vi "Configure Bank Definitions.vi"(8 "error in (no error)":errorcluster, 11 "DIG_IO in":refnum<class "DIG_IO.lvclass">) -> (0 "error out":errorcluster, 3 "DIG_IO out":refnum<class "DIG_IO.lvclass">)   [LabVIEW 2019, in "DIG_IO.lvlib" / "DIG_IO.lvclass"]
uses:
  Library/DIG_IO.lvclass
  Library/DIG_IO.lvclass/DIG_IO.ctl
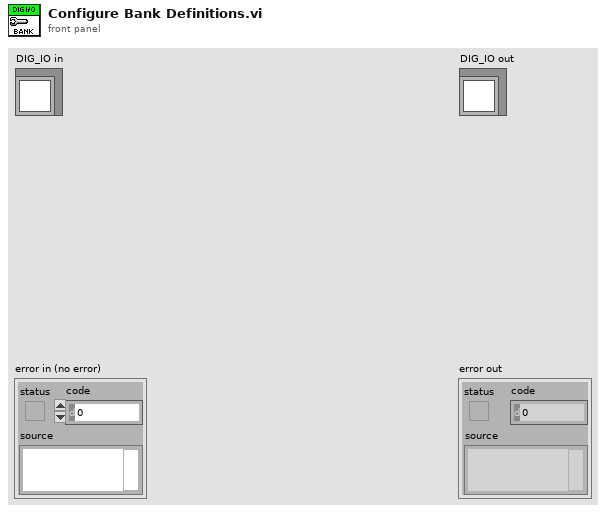
[diagram p1: front panel]
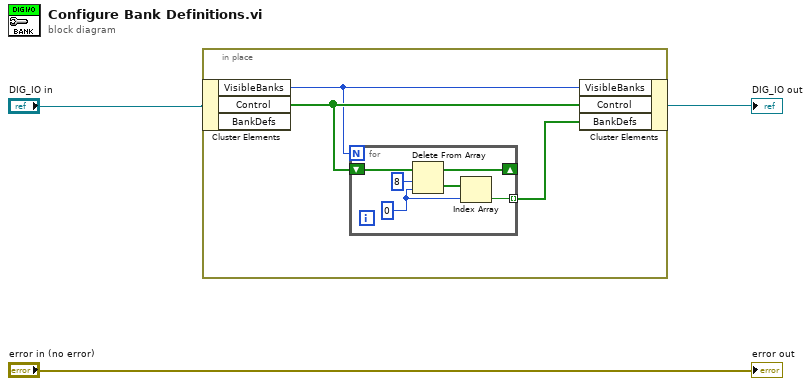
[diagram p0: block diagram]
diagram:
  n1 = in-place {
    n2 = in-place-cluster #1("DIG_IO in") -> ("VisibleBanks"=w5:u8, "Control"=w6:bool[])  [unwired: 1 out]
    n3 = for {
      N: w5 -> [_]
      tunnel: [w7] -> w4 mode=indexing
      shift-right: [w11] -> _
      shift-left: w6 -> [w12]
      w8 = 0 ("index")
      n4 = Delete From Array(array=w12, length=8, index=w8) -> (deleted portion=w9:bool[], array with subset deleted=w11:bool[])
      n5 = Index Array(array=w9, index=w8) -> (element=w7:bool)
    }
    n6 = in-place-cluster #1("VisibleBanks"=w5, "Control"=w6, "BankDefs"=w4) -> (→"DIG_IO out":refnum<class "DIG_IO.lvclass">)
  }
  "error out" <- "error in (no error)"
